vi "DP-Apply Advanced Options.vi"(0 "DataAcq in":T3, 5 "DP params":T1={"Start (dB)"=0.0, "Stop (dB)"=0.0, "Step (dB)"=0.0, "Ear"=enum."Left", "Mode"=enum."L1 = L2", "f2 freqs (kHz)"=""}, 9 "Advanced options":T4, 11 "error in (no error)":errorcluster) -> (4 "DataAcq out":T3, 15 "error out":errorcluster)   [LabVIEW 2020]
uses:
  Typedefs/DP-Advanced Options.ctl
  Typedefs/DP-DataAcq.ctl
  Typedefs/DP Stimulus Params.ctl
  epl-vi-lib/Utility VIs/Type Defs/Left-Right ring.ctl
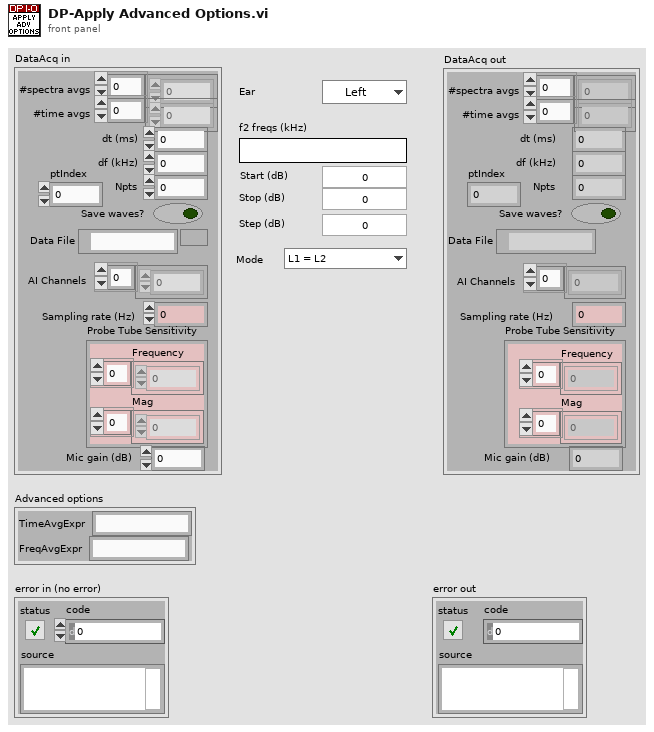
[diagram p1: front panel]
types:
  T1 = typedef "DP Stimulus Params.ctl" = cluster{"Start (dB)":dbl, "Stop (dB)":dbl, "Step (dB)":dbl, "Ear":T2, "Mode":enum16{"L1 = L2", "L1 = L2 + 10 dB"}, "f2 freqs (kHz)":string}
  T2 = typedef "Left-Right ring.ctl" = enum16{"Right", "Left"}
  T3 = typedef "DP-DataAcq.ctl" = cluster{"#spectra avgs":i32[], "#time avgs":i32[], "dt (ms)":dbl, "df (kHz)":dbl, "Npts":i32, "Save waves?":bool, "Data File":path, "AI Channels":u16[], "Sampling rate (Hz)":dbl, "Probe Tube Sensitivity":cluster{"Frequency":dbl[], "Mag":dbl[]}, "Mic gain (dB)":dbl, "ptIndex":i32}
  T4 = typedef "DP-Advanced Options.ctl" = cluster{"TimeAvgExpr":string, "FreqAvgExpr":string}
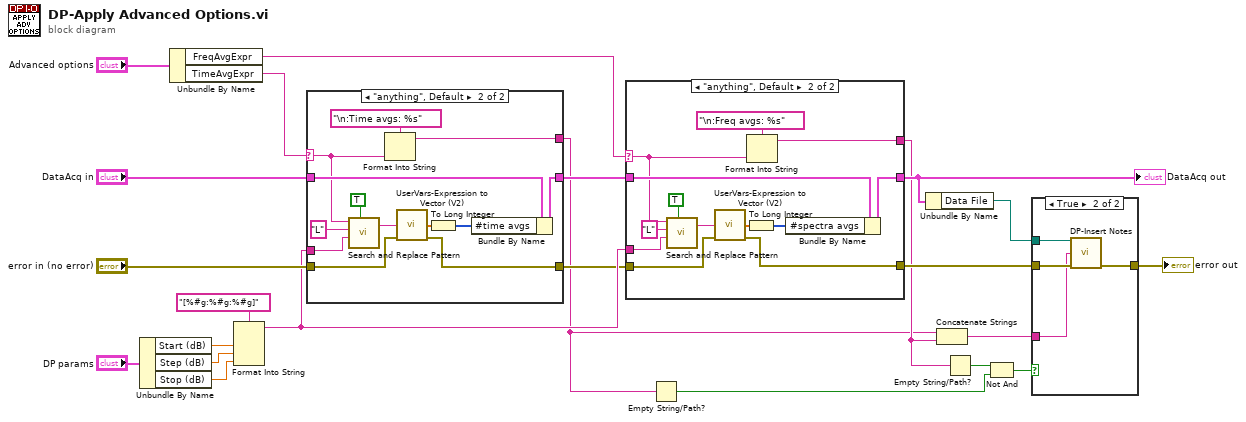
[diagram p0: block diagram]
diagram:
  n1 = Unbundle By Name("DP params") -> ("Start (dB)"=w18:dbl, "Step (dB)"=w17:dbl, "Stop (dB)"=w16:dbl)
  n2 = Unbundle By Name("Advanced options") -> ("FreqAvgExpr"=w11:string, "TimeAvgExpr"=w20:string)
  n3 = Format Into String(format string="[%#g:%#g:%#g]", w18, w17, w16) -> (resulting string=w13:string)  [unwired: 2 in, 1 out]
  n4 = case shown="\"anything\", Default" w20 {
    selector: w20 -> [_ w27]
    tunnel: "DataAcq in" -> [w25 w31]
    tunnel: w13 -> [_ w36]
    tunnel: [w24 w33] -> w12
    tunnel: "error in (no error)" -> [w24 w32]
    tunnel: [w25 w29] -> w14
    tunnel: [_ w26] -> w2
    frame "" {
    }
    frame "anything", Default {
      n5 = call <vilib>:"Search and Replace Pattern.vi"("string"=w27, "regular expression (\"\")"="L" ("regular expression (\"\")"), "replace string (\"\")"=w36, "replace all? (F)"=TRUE) -> ("result string"=w35:string)  [unwired: 1 in, 1 out]
      n6 = Format Into String(format string="\n:Time avgs: %s", w27) -> (resulting string=w26:string)  [unwired: 2 in, 1 out]
      n7 = call "UserVars-Expression to Vector (V2).vi"("Expr"=w35, "error in (no error)"=w32) -> ("Values"=w34:dbl[], "error out"=w33:errorcluster)  [unwired: 12 in]
      n8 = To Long Integer(number=w34) -> (32bit integer=w30:i32[])
      n9 = Bundle By Name(cluster=w31, "#time avgs"=w30) -> (w29:T3)
    }
  }
  n10 = case shown="\"anything\", Default" w11 {
    selector: w11 -> [_ w42]
    tunnel: w14 -> [w40 w47]
    tunnel: w13 -> [_ w51]
    tunnel: [w39 w48] -> w10
    tunnel: [w40 w45] -> w9
    tunnel: w12 -> [w39 w44]
    tunnel: [_ w41] -> w3
    frame "" {
    }
    frame "anything", Default {
      n11 = call <vilib>:"Search and Replace Pattern.vi"("string"=w42, "regular expression (\"\")"="L" ("regular expression (\"\")"), "replace string (\"\")"=w51, "replace all? (F)"=TRUE) -> ("result string"=w50:string)  [unwired: 1 in, 1 out]
      n12 = call "UserVars-Expression to Vector (V2).vi"("Expr"=w50, "error in (no error)"=w44) -> ("Values"=w49:dbl[], "error out"=w48:errorcluster)  [unwired: 12 in]
      n13 = To Long Integer(number=w49) -> (32bit integer=w46:i32[])
      n14 = Format Into String(format string="\n:Freq avgs: %s", w42) -> (resulting string=w41:string)  [unwired: 2 in, 1 out]
      n15 = Bundle By Name(cluster=w47, "#spectra avgs"=w46) -> (w45:T3)
    }
  }
  "DataAcq out" <- w9
  n16 = Empty String/Path?(string/path=w2) -> (empty?=w6:bool)
  n17 = Unbundle By Name(w9) -> ("Data File"=w8:path)
  n18 = Concatenate Strings(w2, w3) -> (w1:string)
  n19 = Empty String/Path?(string/path=w3) -> (empty?=w7:bool)
  n20 = Not And(1:w6, 2:w7) -> (0:w4:bool)
  n21 = case shown="True" w4 {
    tunnel: w10 -> [w54 w58]
    tunnel: w8 -> [_ w57]
    tunnel: [w54 w56] -> w5
    tunnel: w1 -> [_ w55]
    frame False {
    }
    frame True {
      n22 = call "DP-Insert Notes.vi"("path"=w57, "Notes"=w55, "error in (no error)"=w58) -> ("error out"=w56:errorcluster)  [unwired: 12 in]
    }
  }
  "error out" <- w5
